vi "Version String.vi"() -> (1 "string":string, 3 "String":string)   [LabVIEW 2022 SP3]
doc: "Author: Scott Hannahs <sth@magnet.fsu.edu>\nCopyright 2018 Florida State University, All rights reserved."
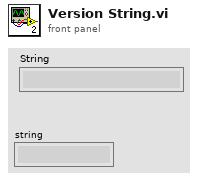
[diagram p1: front panel]
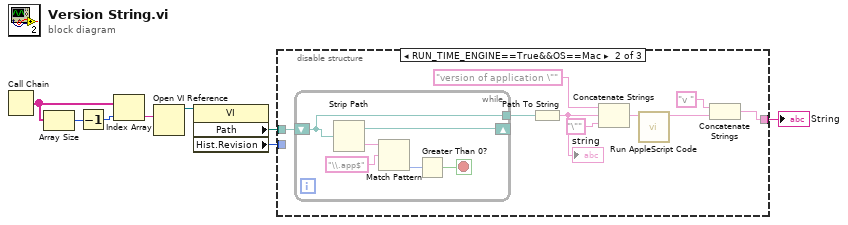
[diagram p0: block diagram]
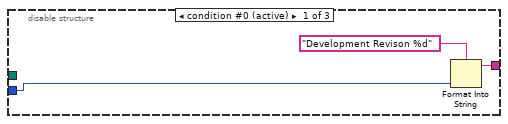
[diagram p2: hidden frame]
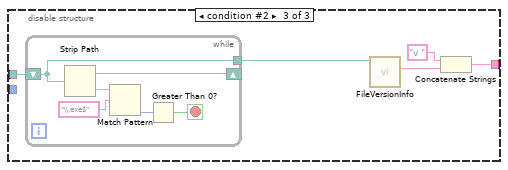
[diagram p3: hidden frame]
diagram:
  n1 = Call Chain() -> (call chain=w5:string[])
  n2 = Array Size(array=w5) -> (size(s)=w7:i32)
  n3 = Decrement(x=w7) -> (x-1=w6:i32)
  n4 = Index Array(array=w5, index=w6) -> (element=w4:string)
  n5 = Open VI Reference(vi path=w4) -> (vi reference=w3:refnum<vi>)  [unwired: 5 in, 1 out]
  n6 = property class="VI"(reference=w3) -> ("Path"=w1:path, "Hist.Revision"=w2:u32)  [unwired: 1 in, 2 out]
  n7 = disable-structure shown="RUN_TIME_ENGINE==True&&OS==Mac" {
    disable-tunnel: [w11 w15 w29] -> w8
    disable-tunnel: w2 -> [w9 _ _]
    disable-tunnel: w1 -> [_ w12 w28]
    frame condition #0 (active) {
      n8 = Format Into String(format string="Development Revison %d", w9) -> (resulting string=w11:string)  [unwired: 2 in, 1 out]
    }
    frame condition #1 {
      n9 = while {
        shift-right: [w26] -> _
        shift-left: w12 -> [w25]
        tunnel: [w25] -> w13
        stop <- w21 stop-if-true
        n10 = Strip Path(path=w25) -> (stripped path=w26:path, name=w22:string)
        n11 = Match Pattern(string=w22, regular expression="\\.app$") -> (offset past match=w24:i32)  [unwired: 1 in, 3 out]
        n12 = Greater Than 0?(x=w24) -> (x > 0?=w21:bool)
      }
      n13 = Path To String(path=w13) -> (string=w18:string)
      "string" <- w18
      n14 = Concatenate Strings("version of application \"", w18, "\"") -> (w20:string)
      n15 = call <vilib>:"Run AppleScript Code.vi"("input string"=w20) -> ("Results"=w16:string)  [unwired: 8 in, 2 out]
      n16 = Concatenate Strings("v ", w16) -> (w15:string)
    }
    frame condition #2 {
      n17 = while {
        shift-right: [w37] -> _
        shift-left: w28 -> [w36]
        tunnel: [w36] -> w27
        stop <- w32 stop-if-true
        n18 = Strip Path(path=w36) -> (stripped path=w37:path, name=w33:string)
        n19 = Match Pattern(string=w33, regular expression="\\.exe$") -> (offset past match=w35:i32)  [unwired: 1 in, 3 out]
        n20 = Greater Than 0?(x=w35) -> (x > 0?=w32:bool)
      }
      n21 = call <vilib>:"FileVersionInfo.vi"("Application Path in"=w27) -> ("File Version Info"=w30:string)  [unwired: 7 in, 3 out]
      n22 = Concatenate Strings("v " ("string"), w30) -> (w29:string)
    }
  }
  "String" <- w8
